vi "Main.vi"(5 "Amplitude (V) :":dbl=5.0 min=-1000000000.0 max=1000000000.0 format="%#_13g", 11 "Error_In":errorcluster) -> (0 "Analog_Waveform":waveform(dbl)(graph)={"t0"=timestamp(0 s since 1904-01-01), "dt"=1e-06, "Y"=array[5000 elements]} caption="Analog Waveform", 3 "Min_Peak_Point":dbl caption="Min Peak Point" format="%.3f V", 4 "Digital_Waveform":digitaldata(graph) caption="Digital Waveform", 6 "Rise_Time (s)":dbl caption="Rise Time (s)" format="%#_6ps", 8 "Fall_Time (s)":dbl caption="Fall Time (s)" format="%#_6ps", 14 "Max_Peak_Point":dbl caption="Max Peak Point" format="%.3f V", 15 "Error_Out":errorcluster)   [LabVIEW 2023]
doc: "This VI is the main VI which communicate with other SubVIs and Displays the output."
panel:
  # "Digitize the Signal"
  # "NOTE: Enter the Amplitude Value to get the Analog waveform, Digital waveform and parameters of the wavfeform"
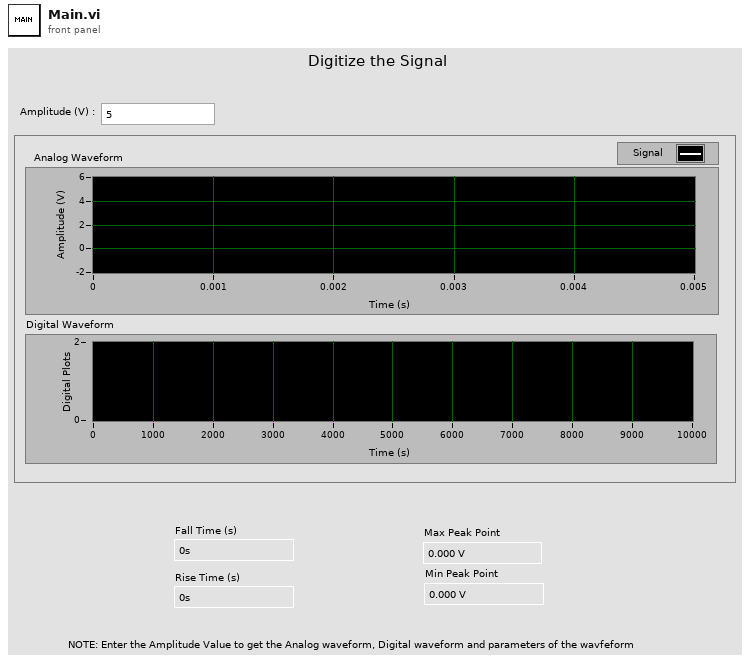
[diagram p1: front panel]
types:
  T1 = enum16{"Left Button", "Center Button", "Right Button", "Window Close"}
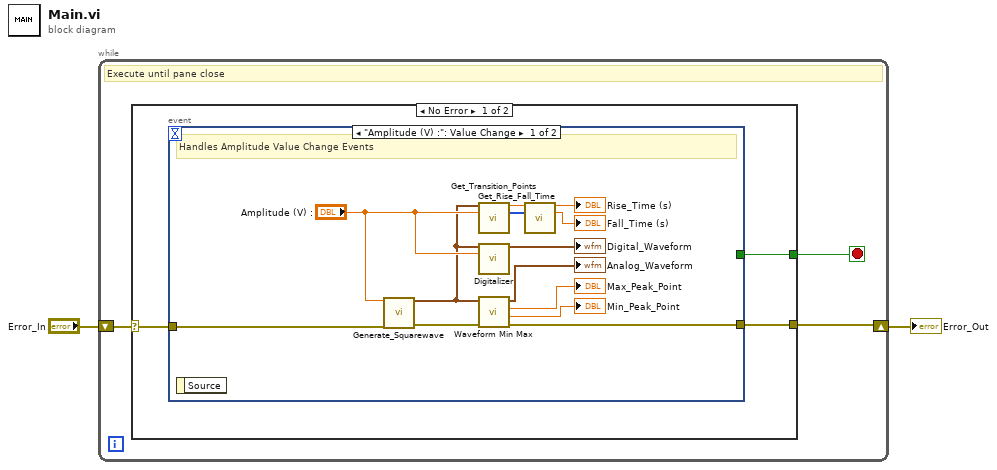
[diagram p0: block diagram]
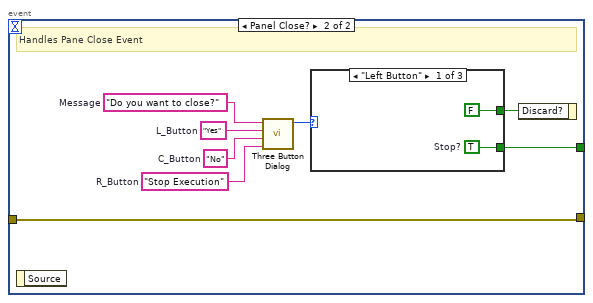
[diagram p2: hidden frame]
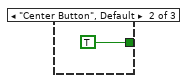
[diagram p3: hidden frame]
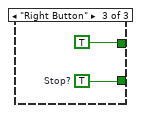
[diagram p4: hidden frame]
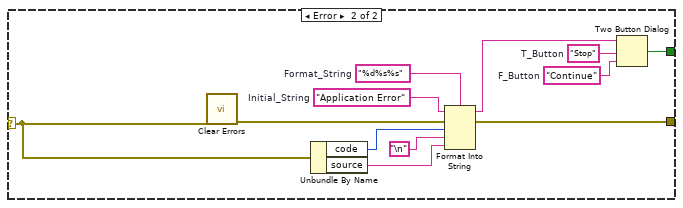
[diagram p5: hidden frame]
diagram:
  n1 = while {
    shift-right: [w3] -> w1
    shift-left: "Error_In" -> [w4]
    stop <- w5 stop-if-true
    # "Execute until pane close"
    n2 = case shown="No Error" w4 {
      selector: w4 -> [w7 w39]
      tunnel: [w8 w35] -> w5
      tunnel: [w6 w40] -> w3
      frame No Error {
        n3 = event shown="[0] \"Amplitude (V) :\": Value Change" {
          selector: _ -> [_ _]
          dyn-events: _ -> [_ _]
          timeout: _ -> [_ _]
          tunnel: [_ w23] -> w8
          tunnel: w7 -> [w16 w22]
          tunnel: [w15 w22] -> w6
          event "Amplitude (V) :": Value Change {
            # "Handles Amplitude Value Change Events"
            n4 = event-data() -> ()  [unwired: 1 in, 1 out]
            n5 = call "Generate_Squarewave.vi"("Amplitude(V)"="Amplitude (V) :", "Error_In"=w16) -> ("Waveform_Out"=w10:waveform(dbl), "Error_Out"=w19:errorcluster)  [unwired: 12 in]
            n6 = call "Get_Transition_Points.vi"("Analog_Waveform"=w10, "Amplitude (V)"="Amplitude (V) :") -> ("dt"=w12:dbl, "Transition_Points"=w11:i32[])  [unwired: 12 in]
            n7 = call "Digitalizer.vi"("Analog_Waveform"=w10, "Amplitude (V)"="Amplitude (V) :") -> ("Digital_Waveform"=→"Digital_Waveform":digitaldata)  [unwired: 13 in]
            n8 = call <vilib>:"Waveform Min Max.vi"("error in (no error)"=w19, "waveform in"=w10) -> ("error out"=w15:errorcluster, "Y min"=→"Min_Peak_Point":dbl, "Y max"=→"Max_Peak_Point":dbl, "waveform out"=→"Analog_Waveform":waveform(dbl))  [unwired: 4 in, 2 out]
            n9 = call "Get_Rise_Fall_Time.vi"("dt"=w12, "Transition_Points"=w11) -> ("Rise_Time (s)"=→"Rise_Time (s)":dbl, "Fall_Time (s)"=→"Fall_Time (s)":dbl)  [unwired: 12 in]
          }
          event Panel Close? {
            w26 = "Stop Execution"  # R_Button
            w27 = "No"  # C_Button
            w28 = "Yes"  # L_Button
            w29 = "Do you want to close?"  # Message
            # "Handles Pane Close Event"
            n10 = event-data() -> ()  [unwired: 1 in, 1 out]
            n11 = call <vilib>:"Three Button Dialog.vi"("Right Button Text (\"Cancel\")"=w26, "Center Button Text (\"No\")"=w27, "Left Button Text (\"Yes\")"=w28, "message"=w29) -> ("Which Button?"=w25:T1)  [unwired: 7 in]
            n12 = case shown="\"Left Button\"" w25 {
              tunnel: [FALSE TRUE TRUE] -> w24
              tunnel: [w30 _ w34] -> w23
              frame "Left Button" {
                w30 = TRUE  # Stop?
              }
              frame "Center Button", Default {
              }
              frame "Right Button" {
                w34 = TRUE  # Stop?
              }
            }
            n13 = event-data("Discard?"=w24) -> ()  [unwired: 1 in, 1 out]
          }
        }
      }
      frame Error {
        w42 = "%d%s%s"  # Format_String
        w43 = "Application Error"  # Initial_String
        w44 = "Stop"  # T_Button
        w45 = "Continue"  # F_Button
        n14 = call <vilib>:"Clear Errors.vi"("error in (no error)"=w39) -> ("error out"=w38:errorcluster)  [unwired: 5 in, 1 out]
        n15 = Unbundle By Name(w39) -> ("code"=w37:i32, "source"=w36:string)
        n16 = Format Into String(format string=w42, initial string=w43, error in=w38, w37, "\n", w36) -> (resulting string=w46:string, error out=w40:errorcluster)
        n17 = Two Button Dialog(message=w46, 1:w45, 2:w44) -> (T button?=w35:bool)
      }
    }
  }
  "Error_Out" <- w1
